vi "PPSU TDK Lambda 2.0.vi"(8 "error in (no error)":errorcluster) -> (0 "error out":errorcluster)   [LabVIEW 2022 SP3]
uses:
  Controls/FGV Read write.ctl
  Controls/ppsu enum.ctl
  SO-Global.vi
panel:
  out "ACKNOWLEDEMENT":string
  out "?":bool
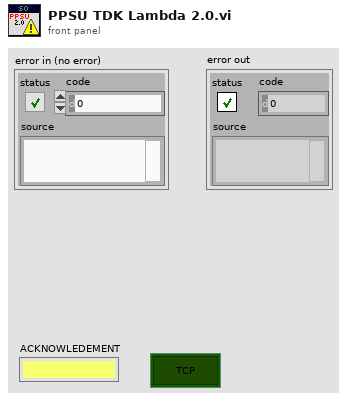
[diagram p1: front panel]
types:
  T1 = typedef "FGV Read write.ctl" = enum16{"Write", "Read"}
  T2 = cluster{"PPSU Actual Voltage ":string, "PPSU Actual Current ":string, "PPSU update Voltage ":dbl, "PPSU Voltage Update":bool, "PPSU Health":bool, "PPSU loop refresh":bool, "PPSU FAULT REGISTER":cluster{"[0]":bool, "[1]":bool, "[2]":bool, "[3]":bool, "[4]":bool, "[5]":bool, "[6]":bool, "[7]":bool, "[8]":bool}, "PPSU STATUS REGISTER":cluster{"[0]":bool, "[1]":bool, "[2]":bool, "[3]":bool, "[4]":bool, "[5]":bool, "[6]":bool, "[7]":bool, "[8]":bool}, "Time Stamp":timestamp, "PPSU FAULT BIT":string, "PPSU STATUS BIT ":string, "PPSU Output":bool}
  T3 = typedef "ppsu enum.ctl" = enum16{"Initialise", "Open connection", "poll event", "ADR", "OVP", "UVL", "VOLTAGE", "CURENT", "OUT ", "Ramp voltage", "FOLD", "save setting", "recall setting", "data log", "stop", "out update", "Internal Ramp", "Internal OFF", "External Ramp", "External ON"}
  T4 = cluster{"Start DAQ":bool, "Stop DAQ":bool, "Start DataLog":bool, "Stop Datalog":bool, "Restart Datalog ":bool, "Exit":bool, "Datalog Title":string, "LCC IP Address:":string}
  T5 = cluster{"START PPSU":bool, "PPSU  Set Current":string, "PPSU Set  Voltage":string, "PPSU OVP":string, "PPSU UVL":string, "PPSU Out":bool, "PPSU Fold":bool, "PPSU Current boolean":bool, "PPSU VOLTAGE bloolean":bool, "Ramp Time":dbl, " External Switch ":bool, " Internal Switch ":bool, "PPSU IP":string}
  T6 = cluster{"[0]":bool, "[1]":bool, "[2]":bool, "[3]":bool, "[4]":bool, "[5]":bool, "[6]":bool, "[7]":bool, "[8]":bool}
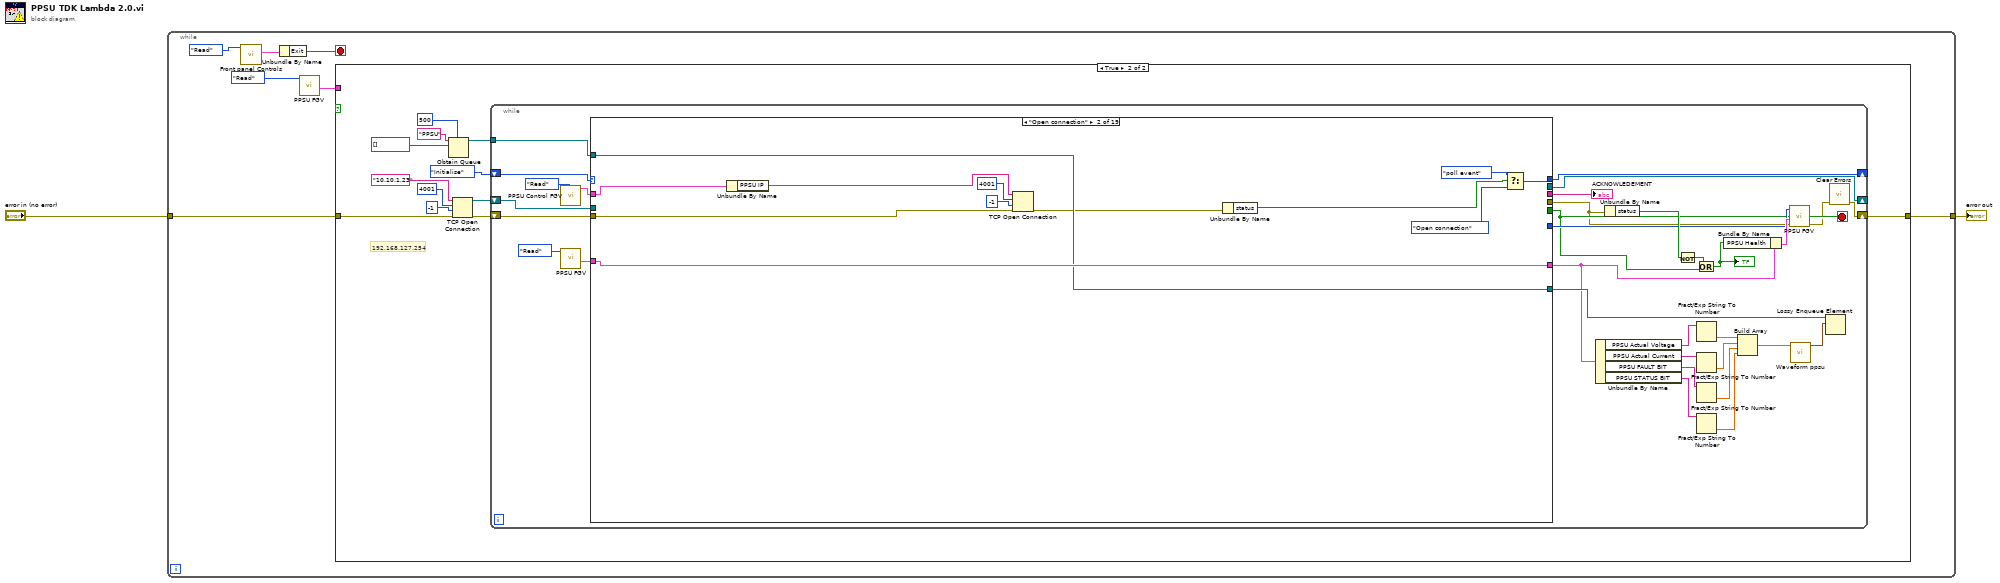
[diagram p0: block diagram]
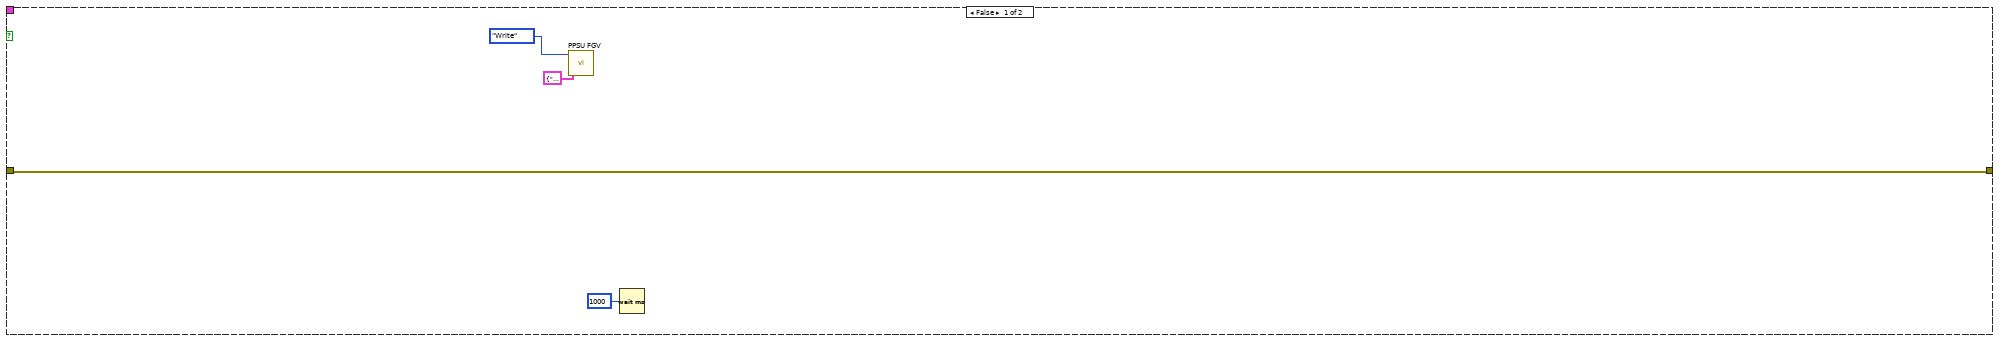
[diagram p2: hidden frame]
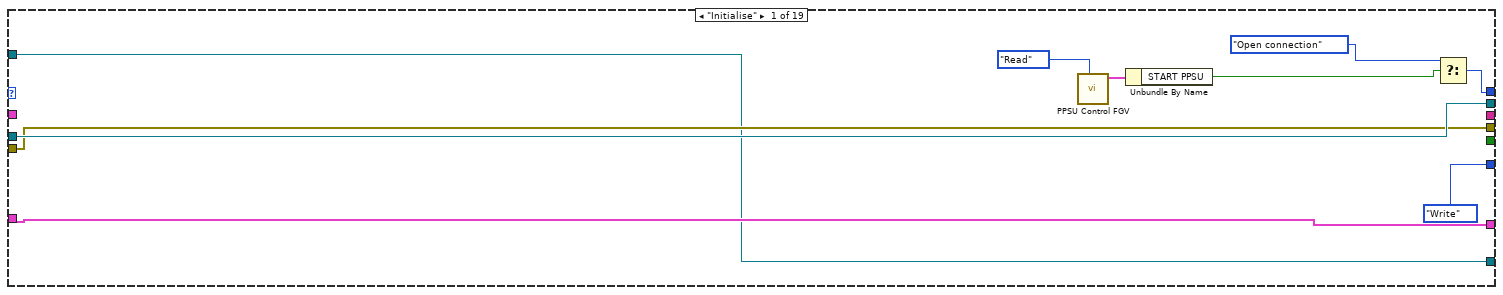
[diagram p3: hidden frame]
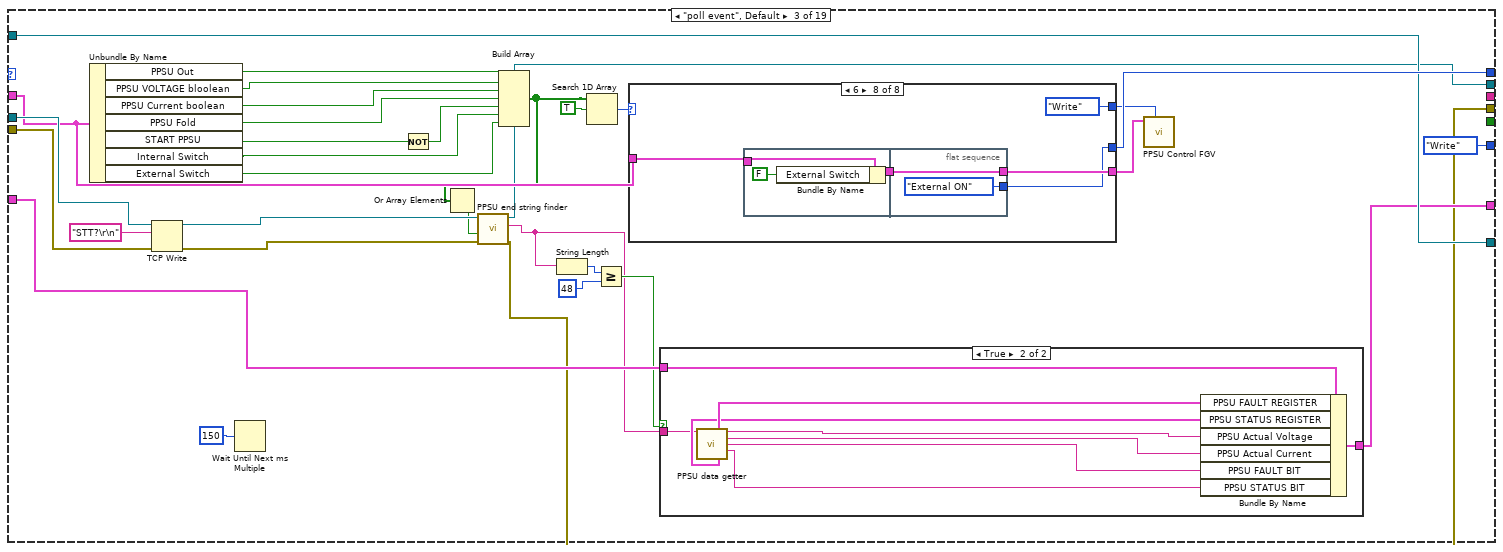
[diagram p4: hidden frame]
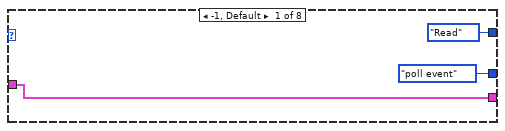
[diagram p6: hidden frame]
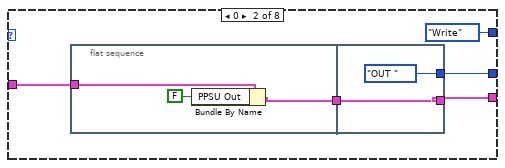
[diagram p7: hidden frame]
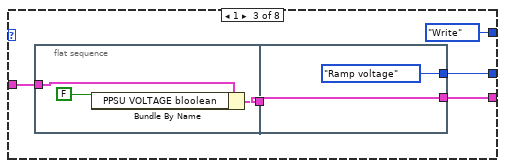
[diagram p8: hidden frame]
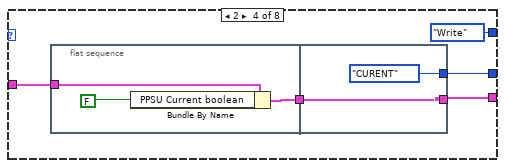
[diagram p9: hidden frame]
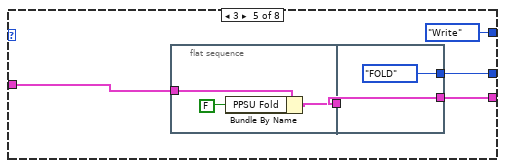
[diagram p10: hidden frame]
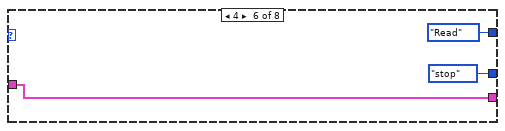
[diagram p11: hidden frame]
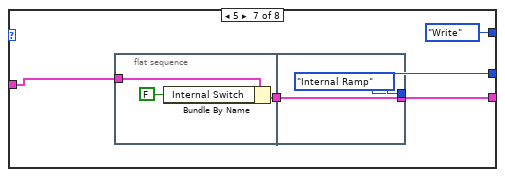
[diagram p12: hidden frame]
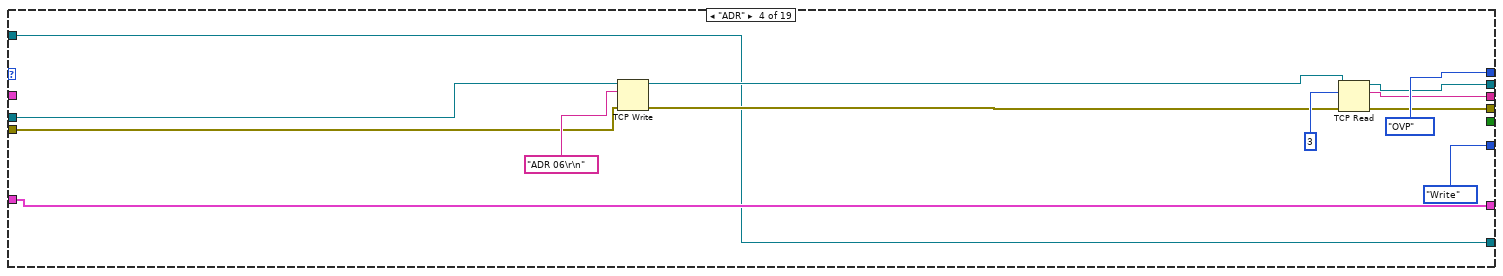
[diagram p13: hidden frame]
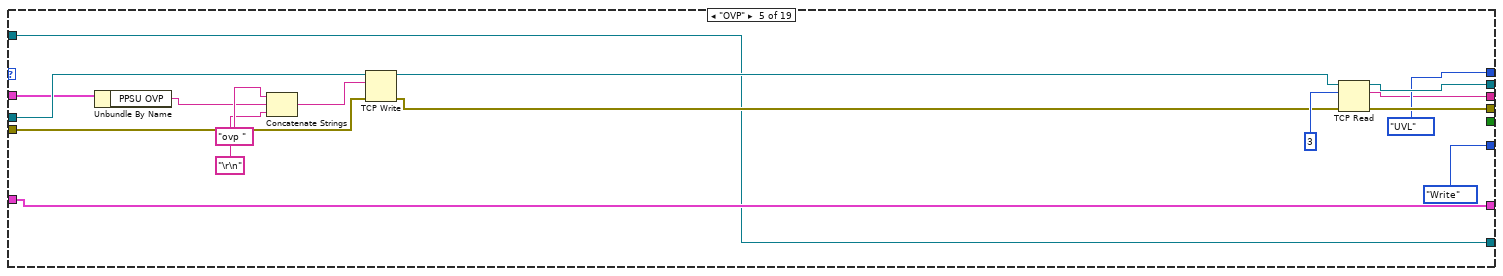
[diagram p14: hidden frame]
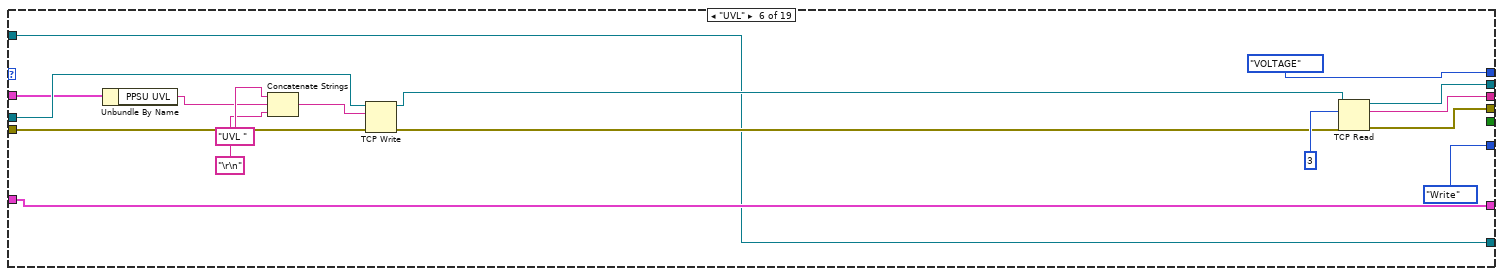
[diagram p15: hidden frame]
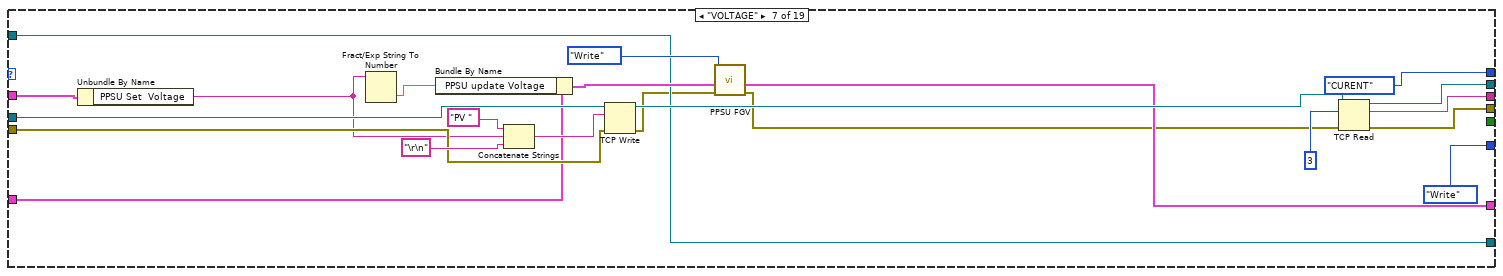
[diagram p16: hidden frame]
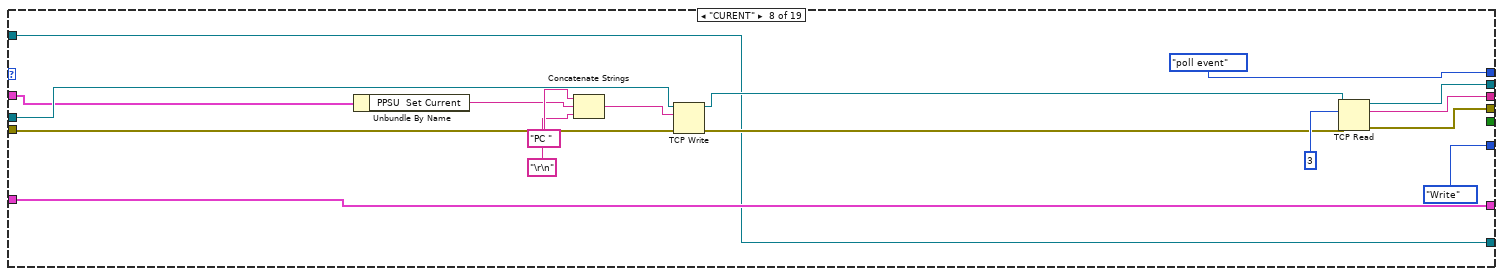
[diagram p17: hidden frame]
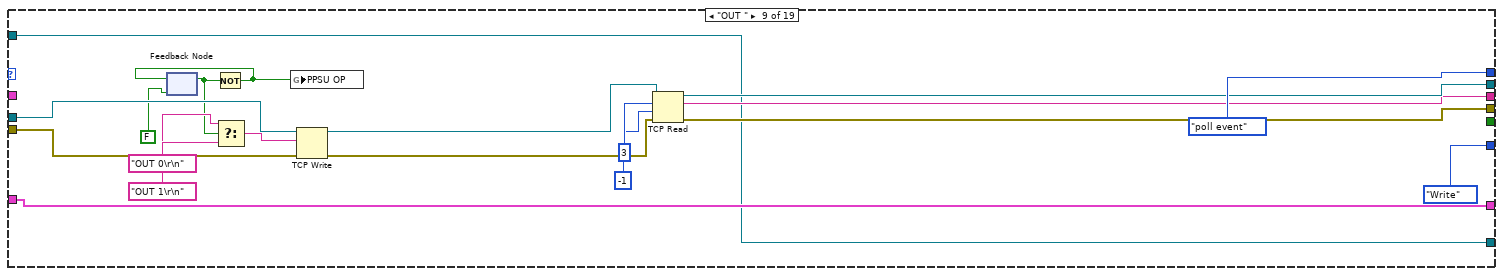
[diagram p18: hidden frame]
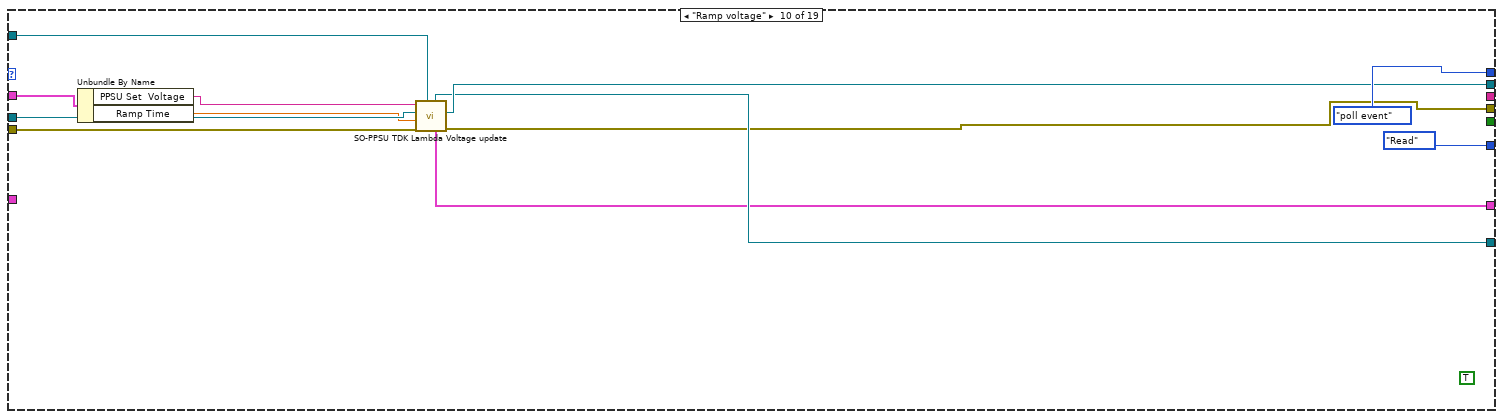
[diagram p19: hidden frame]
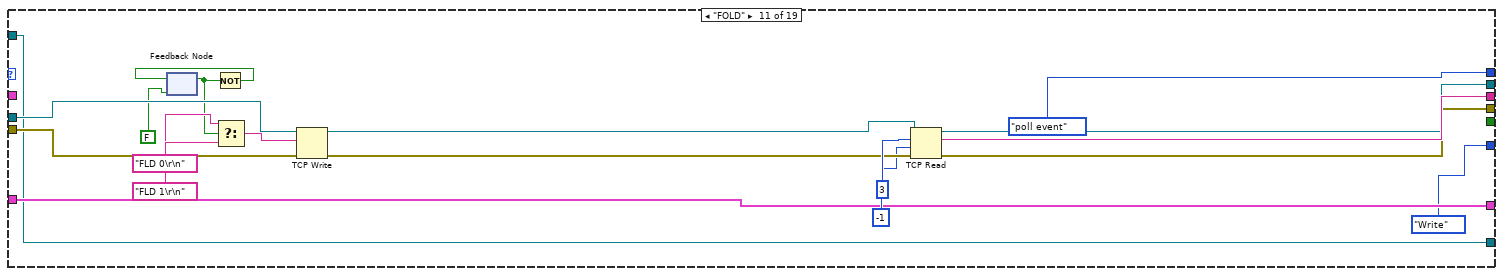
[diagram p20: hidden frame]
diagram:
  n1 = while {
    tunnel: "error in (no error)" -> [w7]
    tunnel: [w3] -> w1
    stop <- w4 stop-if-true
    n2 = call "Front panel Controls.vi"("Write/Read"=FGV_Read_write."Read") -> ("Front Panel Control (R)"=w8:T4)  [unwired: 9 in, 1 out]
    n3 = Unbundle By Name(w8) -> ("Exit"=w4:bool)
    n4 = call "PPSU FGV.vi"("Write/Read"=FGV_Read_write."Read") -> ("PPSU (R)"=w5:T2)  [unwired: 9 in, 1 out]
    n5 = case shown="True" {
      selector: _ -> [_ _]
      tunnel: w7 -> [w13 w24]
      tunnel: [w13 w14] -> w3
      tunnel: w5 -> [_ _]
      frame False {
        n6 = call "PPSU FGV.vi"("PPSU (W)"=T2 {"PPSU Actual Voltage "="", "PPSU Actual Current "="", "PPSU update Voltage "=0.0, "PPSU Voltage Update"=FALSE, "PPSU Health"=FALSE, "PPSU loop refresh"=FALSE, "PPSU FAULT REGISTER"={"[0]"=FALSE, "[1]"=FALSE, "[2]"=FALSE, "[3]"=FALSE, "[4]"=FALSE, "[5]"=FALSE, "[6]"=FALSE, "[7]"=FALSE, "[8]"=FALSE}, "PPSU STATUS REGISTER"={"[0]"=FALSE, "[1]"=FALSE, "[2]"=FALSE, "[3]"=FALSE, "[4]"=FALSE, "[5]"=FALSE, "[6]"=FALSE, "[7]"=FALSE, "[8]"=FALSE}, "Time Stamp"=timestamp(0 s since 1904-01-01), "PPSU FAULT BIT"="", "PPSU STATUS BIT "="", "PPSU Output"=FALSE}, "Write/Read"=FGV_Read_write."Write") -> ()  [unwired: 8 in, 2 out]
        n7 = Wait (ms)(milliseconds to wait=u32 1000) -> ()  [unwired: 1 out]
      }
      frame True {
        # "192.168.127.254"
        n8 = Obtain Queue(max queue size (-1, unlimited)=500, name (unnamed)="PPSU", element data type=waveform(dbl)[] [] ("AI LOX-LP data")) -> (queue out=w16:refnum<queue>)  [unwired: 2 in, 2 out]
        n9 = TCP Open Connection(address="10.10.1.23", remote port or service name=u16 4001, timeout ms (60000)=-1, error in (no error)=w24) -> (connection ID=w15:refnum<k5>, error out=w20:errorcluster)  [unwired: 1 in]
        n10 = while {
          shift-right: [w55] -> _
          shift-left: w15 -> [w57]
          shift-right: [w45] -> w14
          shift-left: w20 -> [w56]
          shift-right: [w53] -> _
          shift-left: ppsu_enum."Initialise" -> [w54]
          tunnel: w16 -> [w44]
          stop <- w38 stop-if-true
          n11 = call "PPSU Control FGV.vi"("Write/Read"=FGV_Read_write."Read") -> ("PPSU Control out"=w48:T5)  [unwired: 9 in, 1 out]
          n12 = call "PPSU FGV.vi"("Write/Read"=FGV_Read_write."Read") -> ("PPSU (R)"=w46:T2)  [unwired: 9 in, 1 out]
          n13 = case shown="\"Open connection\"" w54 {
            tunnel: w57 -> [w67 _ w111 w197 w212 w230 w251 w269 w289 w301 w319 w334 w345 w355 w359 w371 w379 w393 w412]
            tunnel: w56 -> [w66 w72 w110 w196 w211 w229 w250 w268 w288 w300 w318 w332 w344 w354 w358 w373 w381 w396 w414]
            tunnel: [w67 _ w88 w193 w210 w227 w248 w266 w291 w299 w321 w330 w343 w355 w356 w368 w378 w394 w411] -> w55
            tunnel: [w66 _ w86 w192 w209 w225 w247 w265 w290 w294 w320 w329 w342 w354 w357 w372 w380 w395 w413] -> w27
            tunnel: [w59 w76 w108 ppsu_enum."OVP" ppsu_enum."UVL" ppsu_enum."VOLTAGE" ppsu_enum."CURENT" ppsu_enum."poll event" ppsu_enum."poll event" ppsu_enum."poll event" ppsu_enum."poll event" ppsu_enum."poll event" ppsu_enum."poll event" ppsu_enum."poll event" ppsu_enum."stop" ppsu_enum."Internal OFF" ppsu_enum."poll event" ppsu_enum."External Ramp" ppsu_enum."poll event"] -> w53
            tunnel: [_ _ _ w191 w206 w223 w246 w262 w287 _ w322 w327 w340 _ _ _ _ _ _] -> w52
            tunnel: [_ _ _ _ _ _ _ _ _ _ _ _ _ _ TRUE _ _ _ _] -> w38
            tunnel: w48 -> [_ w71 w99 _ w204 w221 w243 w259 _ w303 _ _ _ _ _ _ _ _ w407]
            tunnel: [w65 w79 w93 w190 w203 w220 w241 w260 w277 w293 w307 w326 w339 w352 w362 w367 w377 w392 w408] -> w42
            tunnel: w46 -> [w65 w79 w92 w190 w203 w220 w240 w260 w277 _ w307 w326 w339 w352 w362 _ w388 w403 _]
            tunnel: w44 -> [w64 w78 w95 w189 w202 w219 w239 w258 w276 w295 w306 w325 w338 w351 w361 w370 w390 w405 w410]
            tunnel: [w64 w78 w95 w189 w202 w219 w239 w258 w276 w296 w306 w325 w338 w351 w361 w369 w390 w405 w409] -> w43
            tunnel: [FGV_Read_write."Write" ("Write/Read") _ FGV_Read_write."Write" ("Write/Read") FGV_Read_write."Write" ("Write/Read") FGV_Read_write."Write" ("Write/Read") FGV_Read_write."Write" ("Write/Read") FGV_Read_write."Write" ("Write/Read") FGV_Read_write."Write" ("Write/Read") FGV_Read_write."Write" ("Write/Read") FGV_Read_write."Read" ("Write/Read") FGV_Read_write."Write" ("Write/Read") FGV_Read_write."Write" ("Write/Read") FGV_Read_write."Write" ("Write/Read") FGV_Read_write."Write" ("Write/Read") FGV_Read_write."Write" ("Write/Read") FGV_Read_write."Read" ("Write/Read") FGV_Read_write."Write" ("Write/Read") FGV_Read_write."Write" ("Write/Read") FGV_Read_write."Write" ("Write/Read")] -> w41
            frame "Initialise" {
              n14 = call "PPSU Control FGV.vi"("Write/Read"=FGV_Read_write."Read") -> ("PPSU Control out"=w62:T5)  [unwired: 9 in, 1 out]
              n15 = Unbundle By Name(w62) -> ("START PPSU"=w58:bool)
              n16 = Select(t=ppsu_enum."Open connection", s=w58) -> (s? t:f=w59:T3)  [unwired: 1 in]
            }
            frame "Open connection" {
              n17 = Unbundle By Name(w71) -> ("PPSU IP"=w70:string)
              n18 = TCP Open Connection(address=w70, remote port or service name=u16 4001, timeout ms (60000)=-1, error in (no error)=w72) -> (error out=w69:errorcluster)  [unwired: 1 in, 1 out]
              n19 = Unbundle By Name(w69) -> ("status"=w68:bool)
              n20 = Select(t=ppsu_enum."poll event", s=w68, f=ppsu_enum."Open connection") -> (s? t:f=w76:T3)
            }
            frame "poll event", Default {
              n21 = Unbundle By Name(w99) -> ("PPSU Out"=w104:bool, "PPSU VOLTAGE bloolean"=w103:bool, "PPSU Current boolean"=w102:bool, "PPSU Fold"=w101:bool, "START PPSU"=w100:bool, "Internal Switch"=w81:bool, "External Switch"=w80:bool)
              n22 = TCP Write(connection ID=w111, data in="STT?\r\n", error in (no error)=w110) -> (connection ID out=w84:refnum<k5>, error out=w85:errorcluster)  [unwired: 1 in, 1 out]
              n23 = Wait Until Next ms Multiple(millisecond multiple=u32 150 ("milliseconds to wait")) -> ()  [unwired: 1 out]
              n24 = Not(x=w100) -> (.not. x?=w105:bool)
              n25 = Build Array(w104, w103, w102, w101, w105, w81, w80) -> (w83:bool[])
              n26 = Or Array Elements(Boolean array=w83) -> (logical OR=w82:bool)
              n27 = call "PPSU end string finder.vi"("error in (no error)"=w85, "stop"=w82, "TCP Network Connection in"=w84) -> ("error out"=w86:errorcluster, "String"=w87:string, "TCP Network Connection out"=w88:refnum<k5>)  [unwired: 6 in]
              n28 = String Length(string=w87) -> (length=w91:i32)
              n29 = Search 1D Array(1D array=w83, element=TRUE) -> (index of element=w107:i32)  [unwired: 1 in]
              n30 = Greater Or Equal?(x=w91, y=48) -> (x >= y?=w89:bool)
              n31 = case shown="6" w107 {
                tunnel: [ppsu_enum."poll event" w129 w139 w149 w159 ppsu_enum."stop" w168 w178] -> w108
                tunnel: w99 -> [w123 w128 w138 w148 w158 w166 w171 w181]
                tunnel: [w123 w127 w136 w147 w157 w166 w170 w180] -> w96
                tunnel: [FGV_Read_write."Read" ("Write/Read") FGV_Read_write."Write" ("Write/Read") FGV_Read_write."Write" ("Write/Read") FGV_Read_write."Write" ("Write/Read") FGV_Read_write."Write" ("Write/Read") FGV_Read_write."Read" ("Write/Read") FGV_Read_write."Write" ("Write/Read") FGV_Read_write."Write" ("Write/Read")] -> w97
                frame -1, Default {
                }
                frame 0 {
                  n32 = flat-sequence {
                    tunnel: w128 -> [w132]
                    tunnel: [w130] -> w126
                    tunnel: [ppsu_enum."OUT "] -> w129
                    tunnel: [w133] -> w127
                    tunnel: w126 -> [w133]
                    frame #0 {
                      n33 = Bundle By Name(cluster=w132, "PPSU Out"=FALSE) -> (w130:T5)
                    }
                    frame #1 {
                    }
                  }
                }
                frame 1 {
                  n34 = flat-sequence {
                    tunnel: w138 -> [w141]
                    tunnel: [w140] -> w137
                    tunnel: [ppsu_enum."Ramp voltage"] -> w139
                    tunnel: [w143] -> w136
                    tunnel: w137 -> [w143]
                    frame #0 {
                      n35 = Bundle By Name(cluster=w141, "PPSU VOLTAGE bloolean"=FALSE ("PPSU Out")) -> (w140:T5)
                    }
                    frame #1 {
                    }
                  }
                }
                frame 2 {
                  n36 = flat-sequence {
                    tunnel: w148 -> [w151]
                    tunnel: [w150] -> w146
                    tunnel: [ppsu_enum."CURENT"] -> w149
                    tunnel: [w153] -> w147
                    tunnel: w146 -> [w153]
                    frame #0 {
                      n37 = Bundle By Name(cluster=w151, "PPSU Current boolean"=FALSE ("status")) -> (w150:T5)
                    }
                    frame #1 {
                    }
                  }
                }
                frame 3 {
                  n38 = flat-sequence {
                    tunnel: w158 -> [w162]
                    tunnel: [w160] -> w156
                    tunnel: [ppsu_enum."FOLD"] -> w159
                    tunnel: [w163] -> w157
                    tunnel: w156 -> [w163]
                    frame #0 {
                      n39 = Bundle By Name(cluster=w162, "PPSU Fold"=FALSE ("status")) -> (w160:T5)
                    }
                    frame #1 {
                    }
                  }
                }
                frame 4 {
                }
                frame 5 {
                  n40 = flat-sequence {
                    tunnel: w171 -> [w175]
                    tunnel: [w174] -> w169
                    tunnel: [w177] -> w170
                    tunnel: w169 -> [w177]
                    tunnel: [ppsu_enum."Internal Ramp"] -> w168
                    frame #0 {
                      n41 = Bundle By Name(cluster=w175, "Internal Switch"=FALSE) -> (w174:T5)
                    }
                    frame #1 {
                    }
                  }
                }
                frame 6 {
                  n42 = flat-sequence {
                    tunnel: w181 -> [w185]
                    tunnel: [w184] -> w179
                    tunnel: [w187] -> w180
                    tunnel: w179 -> [w187]
                    tunnel: [ppsu_enum."External ON"] -> w178
                    frame #0 {
                      n43 = Bundle By Name(cluster=w185, "External Switch"=FALSE) -> (w184:T5)
                    }
                    frame #1 {
                    }
                  }
                }
              }
              n44 = case shown="True" w89 {
                tunnel: [w112 w121] -> w93
                tunnel: w92 -> [w112 w120]
                tunnel: w87 -> [_ w113]
                frame False {
                }
                frame True {
                  n45 = call "PPSU data getter.vi"("data in"=w113) -> ("FAULT"=w119:T6, "Voltage PPSU"=w114:string, "Current PPSU"=w116:string, "Fault"=w117:string, "status"=w115:string, "STATUS"=w118:T6)  [unwired: 8 in, 1 out]
                  n46 = Bundle By Name(cluster=w120, "PPSU FAULT REGISTER"=w119, "PPSU STATUS REGISTER"=w118, "PPSU Actual Voltage"=w114, "PPSU Actual Current"=w116, "PPSU FAULT BIT"=w117, "PPSU STATUS BIT"=w115) -> (w121:T2)
                }
              }
              n47 = call "PPSU Control FGV.vi"("Write/Read"=w97, "PPSU Contol in"=w96) -> ()  [unwired: 8 in, 2 out]
            }
            frame "ADR" {
              n48 = TCP Write(connection ID=w197, data in="ADR 06\r\n", error in (no error)=w196) -> (connection ID out=w195:refnum<k5>, error out=w194:errorcluster)  [unwired: 1 in, 1 out]
              n49 = TCP Read(connection ID=w195, bytes to read=3, error in (no error)=w194) -> (connection ID out=w193:refnum<k5>, data out=w191:string, error out=w192:errorcluster)  [unwired: 2 in]
            }
            frame "OVP" {
              n50 = Unbundle By Name(w204) -> ("PPSU OVP"=w205:string)
              n51 = Concatenate Strings("ovp ", w205, "\r\n" ("string")) -> (w215:string)
              n52 = TCP Write(connection ID=w212, data in=w215, error in (no error)=w211) -> (connection ID out=w208:refnum<k5>, error out=w213:errorcluster)  [unwired: 1 in, 1 out]
              n53 = TCP Read(connection ID=w208, bytes to read=3, error in (no error)=w213) -> (connection ID out=w210:refnum<k5>, data out=w206:string, error out=w209:errorcluster)  [unwired: 2 in]
            }
            frame "UVL" {
              n54 = Unbundle By Name(w221) -> ("PPSU UVL"=w222:string)
              n55 = Concatenate Strings("UVL ", w222, "\r\n" ("string")) -> (w232:string)
              n56 = TCP Write(connection ID=w230, data in=w232, error in (no error)=w229) -> (connection ID out=w228:refnum<k5>, error out=w226:errorcluster)  [unwired: 1 in, 1 out]
              n57 = TCP Read(connection ID=w228, bytes to read=3, error in (no error)=w226) -> (connection ID out=w227:refnum<k5>, data out=w223:string, error out=w225:errorcluster)  [unwired: 2 in]
            }
            frame "VOLTAGE" {
              n58 = Unbundle By Name(w243) -> ("PPSU Set  Voltage"=w245:string)
              n59 = Fract/Exp String To Number(string=w245) -> (number=w237:dbl)  [unwired: 3 in, 1 out]
              n60 = Bundle By Name(cluster=w240, "PPSU update Voltage"=w237) -> (w242:T2)
              n61 = Concatenate Strings("PV " ("string"), w245, "\r\n" ("string")) -> (w253:string)
              n62 = TCP Write(connection ID=w251, data in=w253, error in (no error)=w250) -> (connection ID out=w249:refnum<k5>, error out=w236:errorcluster)  [unwired: 1 in, 1 out]
              n63 = call "PPSU FGV.vi"("error in"=w236, "PPSU (W)"=w242, "Write/Read"=FGV_Read_write."Write") -> ("error out"=w235:errorcluster, "PPSU (R)"=w241:T2)  [unwired: 7 in]
              n64 = TCP Read(connection ID=w249, bytes to read=3, error in (no error)=w235) -> (connection ID out=w248:refnum<k5>, data out=w246:string, error out=w247:errorcluster)  [unwired: 2 in]
            }
            frame "CURENT" {
              n65 = Unbundle By Name(w259) -> ("PPSU  Set Current"=w261:string)
              n66 = Concatenate Strings("PC " ("string"), w261, "\r\n" ("string")) -> (w270:string)
              n67 = TCP Write(connection ID=w269, data in=w270, error in (no error)=w268) -> (connection ID out=w263:refnum<k5>, error out=w267:errorcluster)  [unwired: 1 in, 1 out]
              n68 = TCP Read(connection ID=w263, bytes to read=3, error in (no error)=w267) -> (connection ID out=w266:refnum<k5>, data out=w262:string, error out=w265:errorcluster)  [unwired: 2 in]
            }
            frame "OUT " {
              n69 = feedback #1(FALSE) -> (w283:bool)
              n70 = Not(x=w283) -> (.not. x?=w274:bool)
              n71 = feedback-in #1(w274) -> ()
              n72 = Select(t="OUT 0\r\n", s=w283, f="OUT 1\r\n") -> (s? t:f=w278:string)
              n73 = global write "SO-Global.vi" "PPSU OP"(w274) -> ()
              n74 = TCP Write(connection ID=w289, data in=w278, error in (no error)=w288) -> (connection ID out=w281:refnum<k5>, error out=w280:errorcluster)  [unwired: 1 in, 1 out]
              n75 = TCP Read(connection ID=w281, bytes to read=3, error in (no error)=w280, 9:-1 ("timeout ms (25000)")) -> (connection ID out=w291:refnum<k5>, data out=w287:string, error out=w290:errorcluster)  [unwired: 1 in]
            }
            frame "Ramp voltage" {
              (unwired) TRUE
              n76 = Unbundle By Name(w303) -> ("PPSU Set  Voltage"=w302:string, "Ramp Time"=w297:dbl)
              n77 = call "SO-PPSU TDK Lambda Voltage update.vi"("queue In"=w295, "error In"=w300, "Ramp  time(sec)"=w297, "connection ID"=w301, "Voltage"=w302) -> ("error out"=w294:errorcluster, "connection ID 3"=w299:refnum<k5>, "PPSU OUT PUT"=w293:T2, "queue In 2"=w296:refnum<queue>)  [unwired: 2 in, 1 out]
            }
            frame "FOLD" {
              n78 = feedback #2(FALSE) -> (w308:bool)
              n79 = Not(x=w308) -> (.not. x?=w316:bool)
              n80 = feedback-in #2(w316) -> ()
              n81 = Select(t="FLD 0\r\n", s=w308, f="FLD 1\r\n") -> (s? t:f=w315:string)
              n82 = TCP Write(connection ID=w319, data in=w315, error in (no error)=w318) -> (connection ID out=w313:refnum<k5>, error out=w312:errorcluster)  [unwired: 1 in, 1 out]
              n83 = TCP Read(connection ID=w313, bytes to read=3, error in (no error)=w312, 9:-1 ("timeout ms (25000)")) -> (connection ID out=w321:refnum<k5>, data out=w322:string, error out=w320:errorcluster)  [unwired: 1 in]
            }
            frame "save setting" {
              n84 = TCP Write(connection ID=w334, data in="SAV\r\n", error in (no error)=w332) -> (connection ID out=w333:refnum<k5>, error out=w331:errorcluster)  [unwired: 1 in, 1 out]
              n85 = TCP Read(connection ID=w333, bytes to read=3, error in (no error)=w331) -> (connection ID out=w330:refnum<k5>, data out=w327:string, error out=w329:errorcluster)  [unwired: 2 in]
            }
            frame "recall setting" {
              n86 = TCP Write(connection ID=w345, data in="RCL\r\n", error in (no error)=w344) -> (connection ID out=w347:refnum<k5>, error out=w346:errorcluster)  [unwired: 1 in, 1 out]
              n87 = TCP Read(connection ID=w347, bytes to read=3, error in (no error)=w346) -> (connection ID out=w343:refnum<k5>, data out=w340:string, error out=w342:errorcluster)  [unwired: 2 in]
            }
            frame "data log" {
            }
            frame "stop" {
              n88 = TCP Close Connection(connection ID=w359, error in (no error)=w358) -> (connection ID out=w356:refnum<k5>, error out=w357:errorcluster)  [unwired: 1 in]
            }
            frame "Internal Ramp" {
              n89 = call "SO-PPSU TDK Lambda Voltage update.vi"("queue In"=w370, "error In"=w373, "Ramp  time(sec)"=30.0, "connection ID"=w371, "Voltage"="8") -> ("error out"=w372:errorcluster, "connection ID 3"=w368:refnum<k5>, "PPSU OUT PUT"=w367:T2, "queue In 2"=w369:refnum<queue>)  [unwired: 2 in, 1 out]
            }
            frame "Internal OFF" {
              n90 = TCP Write(connection ID=w379, data in="OUT 0\r\n", error in (no error)=w381) -> (connection ID out=w385:refnum<k5>, error out=w386:errorcluster)  [unwired: 1 in, 1 out]
              n91 = Bundle By Name(cluster=w388, "PPSU Output"=FALSE ("PPSU OP")) -> (w377:T2)
              n92 = TCP Read(connection ID=w385, bytes to read=3, error in (no error)=w386, 9:-1 ("timeout ms (25000)")) -> (connection ID out=w378:refnum<k5>, error out=w380:errorcluster)  [unwired: 1 in, 1 out]
            }
            frame "External ON" {
              n93 = TCP Write(connection ID=w393, data in="OUT 1\r\n", error in (no error)=w396) -> (connection ID out=w400:refnum<k5>, error out=w401:errorcluster)  [unwired: 1 in, 1 out]
              n94 = Bundle By Name(cluster=w403, "PPSU Output"=TRUE ("PPSU OP")) -> (w392:T2)
              n95 = TCP Read(connection ID=w400, bytes to read=3, error in (no error)=w401, 9:-1 ("timeout ms (25000)")) -> (connection ID out=w394:refnum<k5>, error out=w395:errorcluster)  [unwired: 1 in, 1 out]
            }
            frame "External Ramp" {
              n96 = Unbundle By Name(w407) -> ("PPSU Set  Voltage"=w406:string)
              n97 = call "SO-PPSU TDK Lambda Voltage update.vi"("queue In"=w410, "error In"=w414, "Ramp  time(sec)"=30.0, "connection ID"=w412, "Voltage"=w406) -> ("error out"=w413:errorcluster, "connection ID 3"=w411:refnum<k5>, "PPSU OUT PUT"=w408:T2, "queue In 2"=w409:refnum<queue>)  [unwired: 2 in, 1 out]
            }
          }
          "ACKNOWLEDEMENT" <- w52
          n98 = Unbundle By Name(w42) -> ("PPSU Actual Voltage"=w31:string, "PPSU Actual Current"=w30:string, "PPSU FAULT BIT"=w29:string, "PPSU STATUS BIT"=w28:string)
          n99 = Unbundle By Name(w27) -> ("status"=w51:bool)
          n100 = Not(x=w51) -> (.not. x?=w40:bool)
          n101 = Or(x=w40, y=w38) -> (x .or. y?=w39:bool)
          "?" <- w39
          n102 = Fract/Exp String To Number(string=w31) -> (number=w36:dbl)  [unwired: 3 in, 1 out]
          n103 = Fract/Exp String To Number(string=w30) -> (number=w35:dbl)  [unwired: 3 in, 1 out]
          n104 = Fract/Exp String To Number(string=w29) -> (number=w34:dbl)  [unwired: 3 in, 1 out]
          n105 = Fract/Exp String To Number(string=w28) -> (number=w33:dbl)  [unwired: 3 in, 1 out]
          n106 = Bundle By Name(cluster=w42, "PPSU Health"=w39) -> (w50:T2)
          n107 = Build Array(w36, w35, w34, w33) -> (w32:dbl[])
          n108 = call "PPSU FGV.vi"("error in"=w27, "PPSU (W)"=w50, "Write/Read"=w41) -> ("error out"=w26:errorcluster)  [unwired: 7 in, 1 out]
          n109 = call "Waveform ppsu.vi"("Array in"=w32) -> ("Array out"=w37:waveform(dbl)[])  [unwired: 10 in]
          n110 = Lossy Enqueue Element(queue=w43, element=w37) -> ()  [unwired: 1 in, 4 out]
          n111 = call <vilib>:"Clear Errors.vi"("error in (no error)"=w26) -> ("error out"=w45:errorcluster)  [unwired: 5 in, 1 out]
        }
      }
    }
  }
  "error out" <- w1
